vi "Pump Status.vi"(8 "error in (no error)":errorcluster, 11 "Masterflex Settings in":T1={"VISA resource name"="", "Simulated?"=FALSE, "Pump Number"=1.0, "Reverse?"=FALSE} {"Pump Number" min=1.0 max=20.0 step=1.0}) -> (0 "error out":errorcluster, 1 "Connection Error":bool, 2 "Pump On?":enum16{"Off", "On", "Not Initialized"}(ring), 3 "Masterflex Settings out":T1={"VISA resource name"="", "Simulated?"=FALSE, "Pump Number"=1.0, "Reverse?"=FALSE} {"Pump Number" min=1.0 max=20.0 step=1.0})   [LabVIEW 2018, in "Masterflex 7550-30.lvlib"]
uses:
  Masterflex 7550-30.lvlib
  Controls/Settings Cluster.ctl
  <vilib>/Instr/_visa.llb/VISA Flush IO Buffer Mask.ctl
  <vilib>/Instr/_visa.llb/VISA Configure Serial Port (Instr).vi
  <vilib>/regexp/Match Regular Expression.xnode
panel:
  out "Pump Status":string
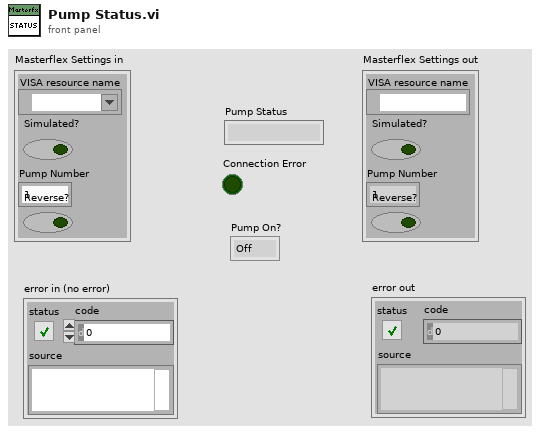
[diagram p1: front panel]
types:
  T1 = typedef "Masterflex 7550-30.lvlib/Settings Cluster.ctl" = cluster{"VISA resource name":refnum<visa-resource-name>, "Simulated?":bool, "Pump Number":dbl, "Reverse?":bool}
  T2 = typedef "VISA Flush IO Buffer Mask.ctl" = u16
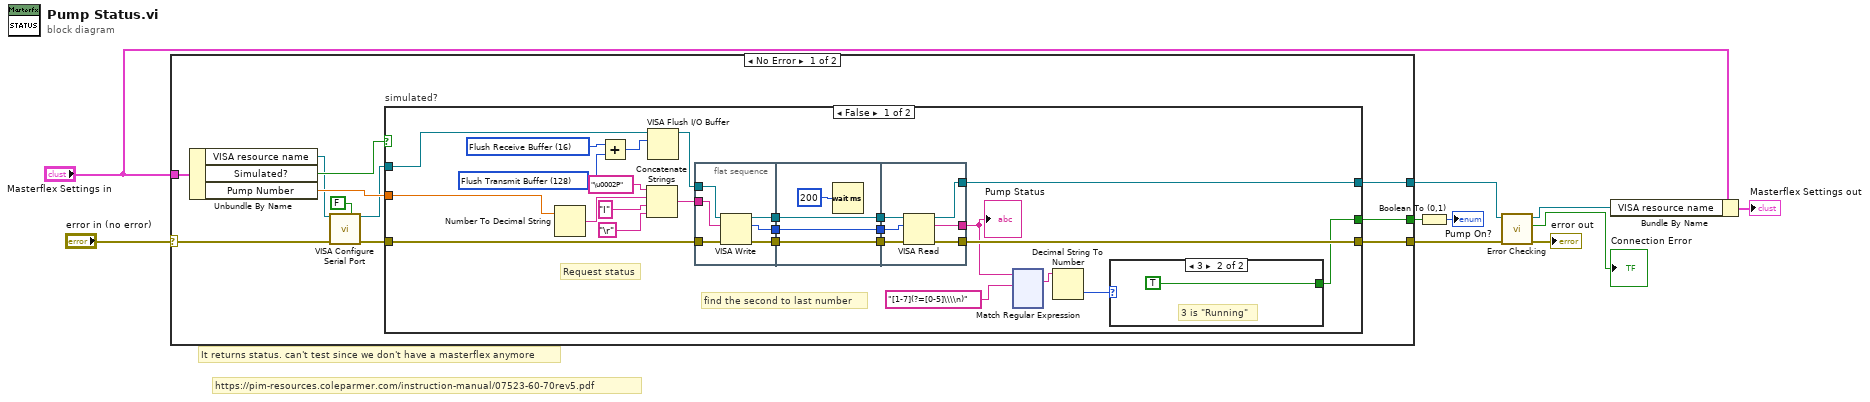
[diagram p0: block diagram]
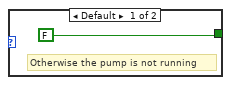
[diagram p2: hidden frame]
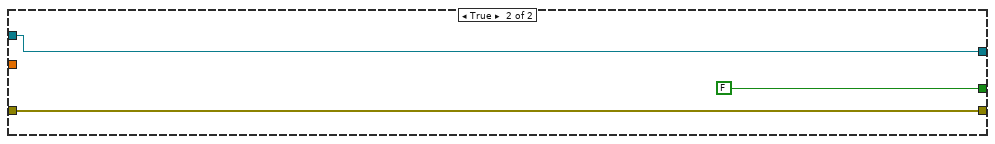
[diagram p3: hidden frame]
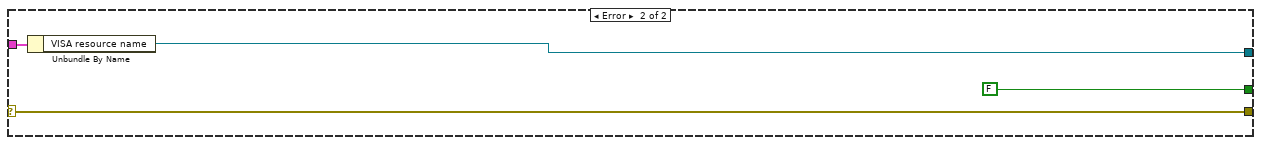
[diagram p4: hidden frame]
diagram:
  # "https://pim-resources.coleparmer.com/instruction-manual/07523-60-70rev5.pdf"
  # "It returns status. can't test since we don't have a masterflex anymore"
  n1 = case shown="No Error" "error in (no error)" {
    selector: "error in (no error)" -> [w14 w185]
    tunnel: [w20 w185] -> w8
    tunnel: "Masterflex Settings in" -> [w19 w183]
    tunnel: [w12 FALSE] -> w2
    tunnel: [w17 w182] -> w7
    frame No Error {
      n2 = Unbundle By Name(w19) -> ("VISA resource name"=w16:refnum<visa-resource-name>, "Simulated?"=w21:bool, "Pump Number"=w18:dbl)
      n3 = call-poly "VISA Configure Serial Port"("VISA resource name"=w16, "Enable Termination\nChar (T)"=FALSE ("Enable Termination\nChar (T)"), "error in (no error)"=w14) -> ("VISA resource name out"=w15:refnum<visa-resource-name>, "error out"=w13:errorcluster)  [unwired: 11 in]
      n4 = case "simulated?" shown="False" w21 {
        tunnel: [w35 w180] -> w20
        tunnel: [w27 w179] -> w17
        tunnel: w18 -> [w43 _]
        tunnel: w13 -> [w37 w180]
        tunnel: w15 -> [w29 w179]
        tunnel: [w22 FALSE] -> w12
        frame False {
          w31 = T2 128 items=["Flush Receive Buffer"=16, "Write Transmit Buffer to Device"=32, "Flush Receive Buffer (No I/O)"=64, "Flush Transmit Buffer"=128] ("Mask")
          w30 = T2 16 items=["Flush Receive Buffer"=16, "Write Transmit Buffer to Device"=32, "Flush Receive Buffer (No I/O)"=64, "Flush Transmit Buffer"=128] ("Mask")
          # "Request status"
          # "find the second to last number"
          n5 = Number To Decimal String(number=w43) -> (decimal integer string=w42:string)  [unwired: 1 in]
          n6 = Add(x=w30, y=w31) -> (x+y=w32:T2)
          n7 = Concatenate Strings("\u0002P" ("string"), w42, "I" ("string"), "\r") -> (w36:string)
          n8 = VISA Flush I/O Buffer(VISA resource name=w29, mask (16)=w32) -> (VISA resource name out=w28:refnum<visa-resource-name>)  [unwired: 1 in, 1 out]
          n9 = flat-sequence {
            tunnel: [w166] -> w39
            tunnel: [w167] -> w38
            tunnel: w37 -> [w163]
            tunnel: w36 -> [w168]
            tunnel: w28 -> [w164]
            tunnel: [w165] -> w34
            tunnel: [w172] -> w41
            tunnel: [w171] -> w40
            tunnel: w39 -> [w172]
            tunnel: w38 -> [w171]
            tunnel: w34 -> [w169]
            tunnel: [w169] -> w33
            tunnel: w41 -> [w178]
            tunnel: w40 -> [w177]
            tunnel: [w174] -> w35
            tunnel: w33 -> [w176]
            tunnel: [w175] -> w25
            tunnel: [w173] -> w27
            frame #0 {
              n10 = VISA Write(VISA resource name=w164, write buffer=w168, error in (no error)=w163) -> (VISA resource name out=w166:refnum<visa-resource-name>, return count=w165:u32, error out=w167:errorcluster)
            }
            frame #1 {
              n11 = Wait (ms)(milliseconds to wait=u32 200) -> ()  [unwired: 1 out]
            }
            frame #2 {
              n12 = VISA Read(VISA resource name=w178, byte count=w176, error in (no error)=w177) -> (VISA resource name out=w173:refnum<visa-resource-name>, read buffer=w175:string, error out=w174:errorcluster)  [unwired: 1 out]
            }
          }
          n13 = xnode "Match Regular Expression"("input string"=w25, "regular expression"="[1-7](?=[0-5]\\\\n)") -> ("whole match"=w24:string)  [unwired: 4 in, 4 out]
          n14 = Decimal String To Number(string=w24) -> (number=w23:i32)  [unwired: 2 in, 1 out]
          n15 = case shown="3" w23 {
            tunnel: [FALSE TRUE] -> w22
            frame Default {
              # "Otherwise the pump is not running"
            }
            frame 3 {
              # "3 is \"Running\""
            }
          }
          "Pump Status" <- w25
        }
        frame True {
        }
      }
    }
    frame Error {
      n16 = Unbundle By Name(w183) -> ("VISA resource name"=w182:refnum<visa-resource-name>)
    }
  }
  n17 = Boolean To (0,1)(Boolean=w2) -> (0, 1=→"Pump On?":i16)
  n18 = call "Error Checking.vi"("error in (no error)"=w8, "VISA resource name"=w7) -> ("error out"=→"error out":errorcluster, "Connection Error"=→"Connection Error":bool, "VISA resource name"=w5:refnum<visa-resource-name>)  [unwired: 7 in]
  n19 = Bundle By Name(cluster="Masterflex Settings in", "VISA resource name"=w5) -> (→"Masterflex Settings out":T1)
